vi "Teleop.vi"(10 "Match Info":T1={"Autonomous Elapsed Seconds"=0.0, "TeleOp Elapsed Seconds"=0.0, "Disabled Elapsed Seconds"=0.0, "Visited Autonomous"=FALSE, "Visited TeleOp"=FALSE, "Visited Disabled"=FALSE, "Autonomous Settings"={"Autonomous Style"=enum."Independent", "VI Refnum"=refnum}}, 11 "Call Context":T2) -> ()   [LabVIEW 2018]
doc: "This VI is called for each enabled TeleOp packet received from the DS. It is typically used to read from joysticks and other inputs and update I/O or setpoints for timed control loops. It should complete and return within 20 milliseconds or risk missing DS packets."
uses:
  <vilib>/Rock Robotics/WPI/DriverStation/WPI_DriverStationDerivedRobotMode.ctl
  <vilib>/Rock Robotics/WPI/DriverStation/WPI_DriverStationMatch Info.ctl
  <vilib>/Rock Robotics/WPI/ThirdParty/Phoenix-LabVIEW/Motor Controller/Controls/CTRE_Phoenix_MotorControl_ControlMode.ctl
  <vilib>/Rock Robotics/WPI/Utilities/WPI_GetSetVariantRefNum.vi
  <vilib>/Rock Robotics/Network Tables/NT Write Boolean.vi
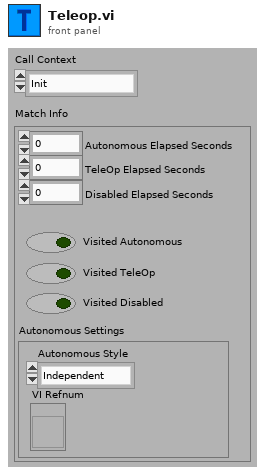
[diagram p1: front panel]
types:
  T1 = typedef "WPI_DriverStationMatch Info.ctl" = cluster{"Autonomous Elapsed Seconds":dbl, "TeleOp Elapsed Seconds":dbl, "Disabled Elapsed Seconds":dbl, "Visited Autonomous":bool, "Visited TeleOp":bool, "Visited Disabled":bool, "Autonomous Settings":cluster{"Autonomous Style":enum16{"Iterative", "Independent"}, "VI Refnum":refnum<vi>}}
  T2 = typedef "WPI_DriverStationDerivedRobotMode.ctl" = enum16{"Init", "Execute", "Stop"}
  T3 = enum16{"Low Ball", "Middle Ball", "High Ball", "High Hatch", "Middle Hatch", "Low Hatch", "Cargo Ball", "Ball Loading Station", "Ball Ground", "Reserve"}
  T4 = typedef "WPI_JoystickDevRef.ctl" = cluster{"Device":T5}
  T5 = typedef "WPI_JoystickDeviceEnum.ctl" = enum16{"USB 0", "USB 1", "USB 2", "USB 3", "USB 4", "USB 5"}
  T6 = cluster{"POVs[0]":i16, "POVs[1]":i16, "POVs[2]":i16, "POVs[3]":i16, "POVs[4]":i16, "POVs[5]":i16, "POVs[6]":i16, "POVs[7]":i16, "POVs[8]":i16}
  T7 = typedef "WPI_MotorControlDeviceRef.ctl" = cluster{"DeviceStatus":errorcluster, "Type":T8, "PWM":cluster{"PWM Channel":T9, "DeadBand":T10}, "CAN":cluster{"Device Number":u8, "SetOutput VI Ref":variant, "GetOutput VI Ref":variant, "Enable VI Ref":variant, "Disable VI Ref":variant, "Data":variant}, "Invert":bool, "DIO PWM":cluster{"PWM \"Enable\" Channel":T9, "DIOChannel":T11, "PWM Rate":dbl}}
  T8 = typedef "WPI_MotorControlType.ctl" = enum16{"PWM", "CAN", "DIO PWM"}
  T9 = typedef "FPGA_DIOPWMChannel.ctl" = enum8{"PWM 0", "PWM 1", "PWM 2", "PWM 3", "PWM 4", "PWM 5", "PWM 6", "PWM 7", "PWM 8", "PWM 9", "PWM MXP 0", "PWM MXP 1", "PWM MXP 2", "PWM MXP 3", "PWM MXP 4", "PWM MXP 5", "PWM MXP 6", "PWM MXP 7", "PWM MXP 8", "PWM MXP 9", "Invalid"}
  T10 = typedef "WPI_PWMDeadband.ctl" = cluster{"Name":string, "maxPositivePwm":i32, "minPositivePwm":i32, "centerPwm":i32, "maxNegativePwm":i32, "minNegativePwm":i32, "angularRange":u16}
  T11 = typedef "FPGA_DIOChannel.ctl" = enum8{"DIO 0", "DIO 1", "DIO 2", "DIO 3", "DIO 4", "DIO 5", "DIO 6", "DIO 7", "DIO 8", "DIO 9", "DIO MXP 0", "DIO MXP 1", "DIO MXP 2", "DIO MXP 3", "DIO MXP 4", "DIO MXP 5", "DIO MXP 6", "DIO MXP 7", "DIO MXP 8", "DIO MXP 9", "DIO MXP 10", "DIO MXP 11", "DIO MXP 12", "DIO MXP 13", "DIO MXP 14", "DIO MXP 15", "SPI Port CS1", "SPI Port CS2", "SPI Port CS3", "SPI Port MISO", "SPI Port MOSI", "Invalid"}
  T12 = typedef "CTRE_Phoenix_MotorControl_ControlMode.ctl" = u16
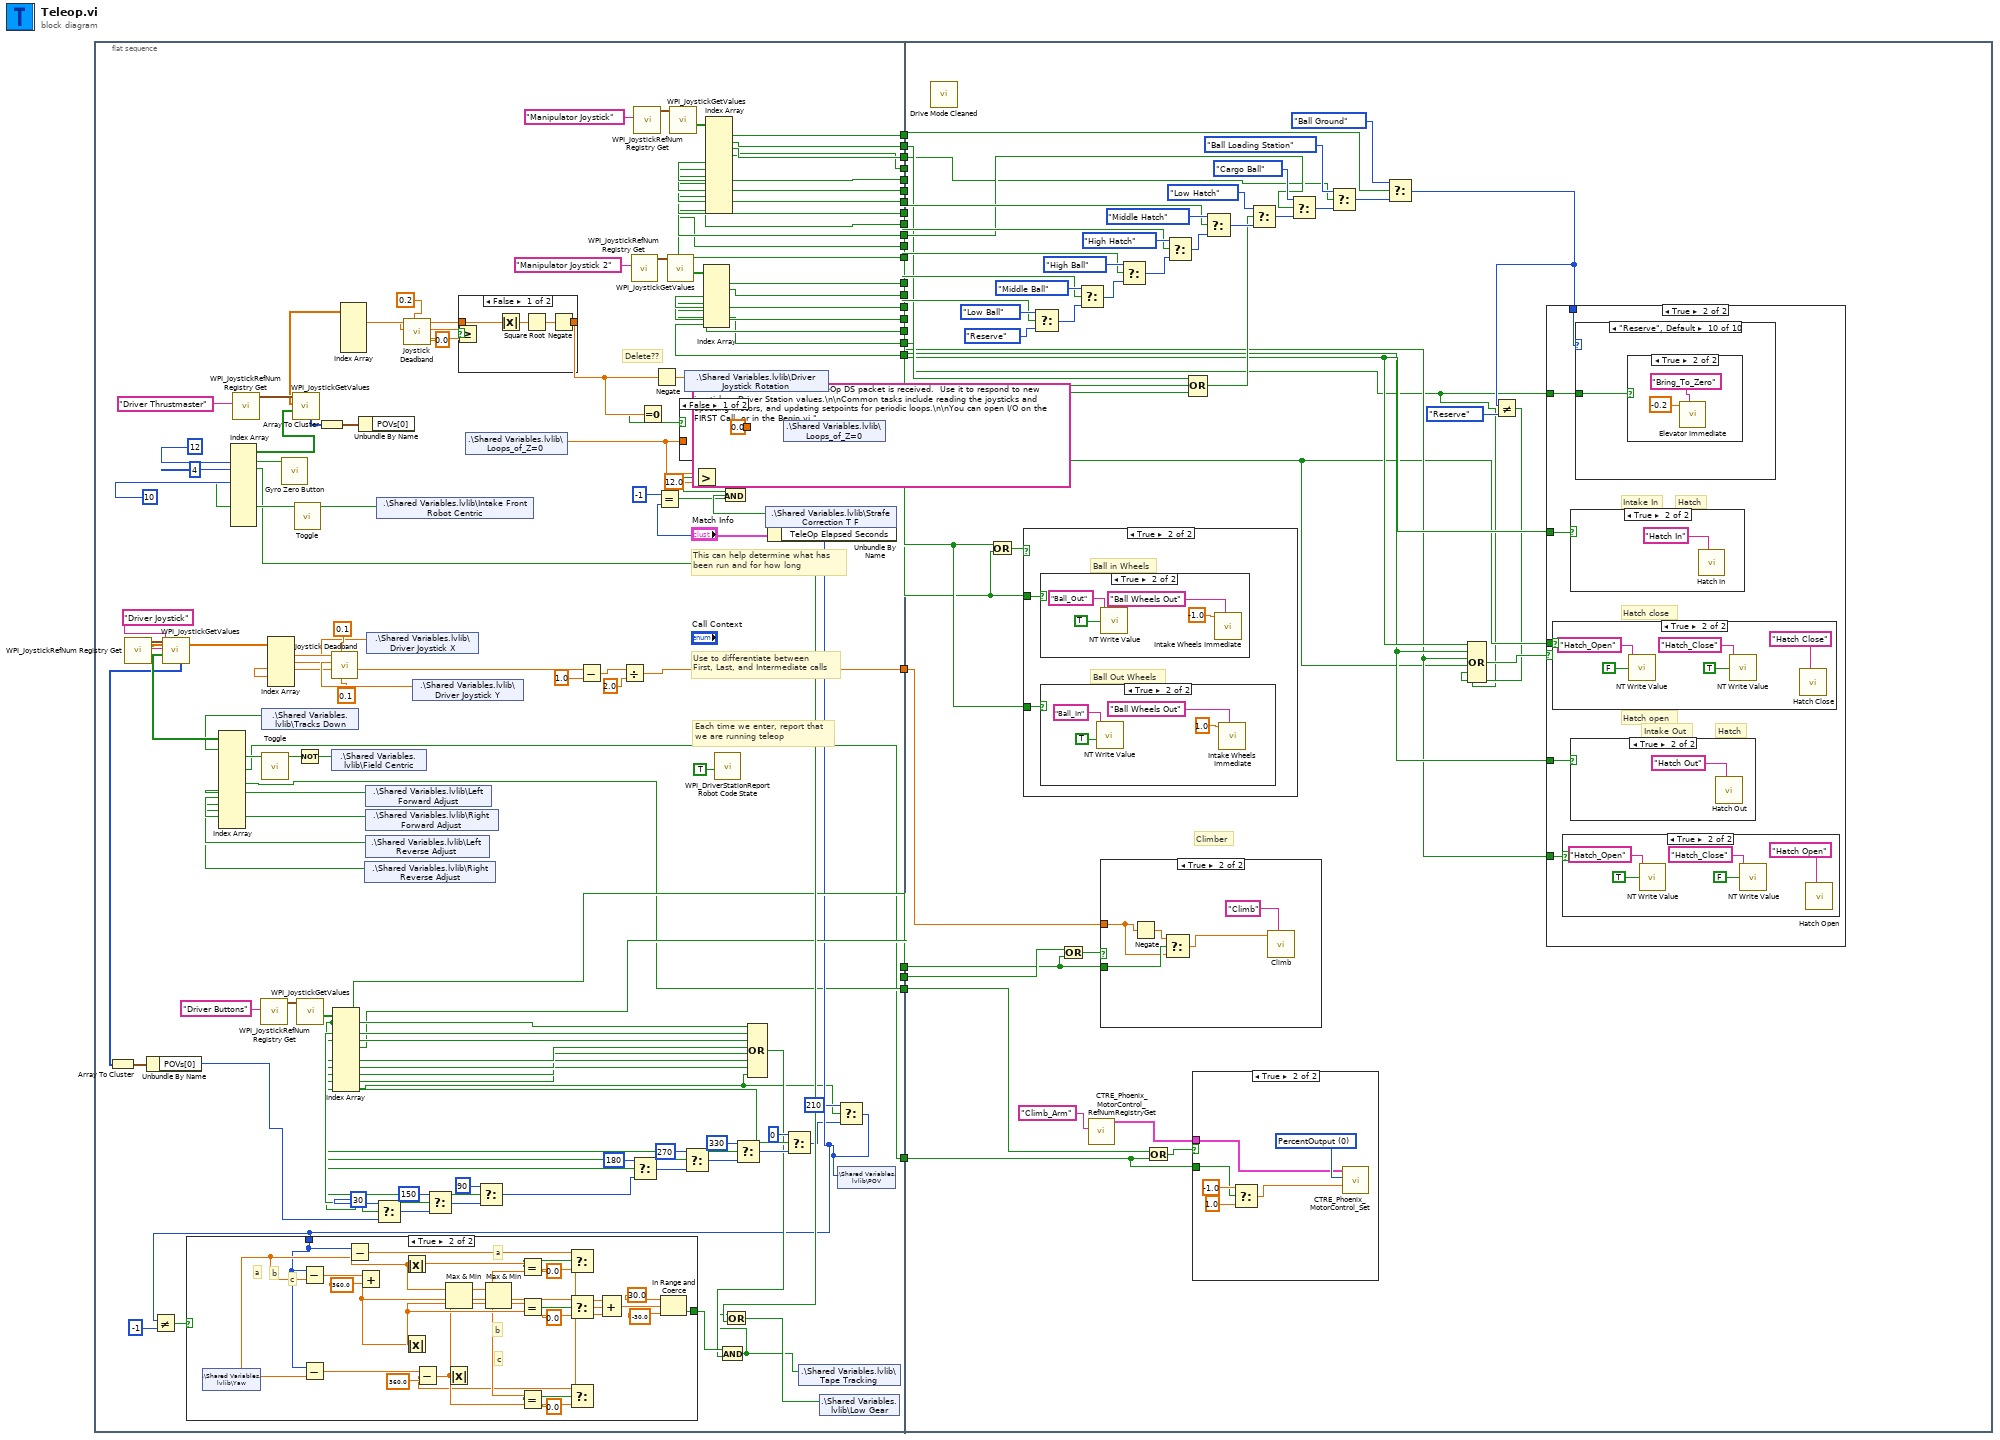
[diagram p0: block diagram]
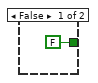
[diagram p2: hidden frame]
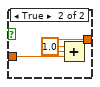
[diagram p3: hidden frame]
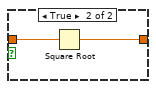
[diagram p4: hidden frame]
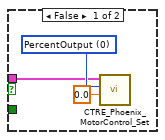
[diagram p5: hidden frame]
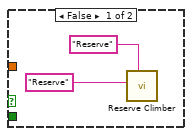
[diagram p6: hidden frame]
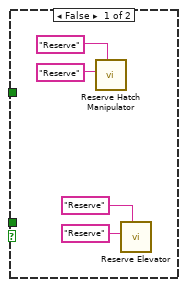
[diagram p7: hidden frame]
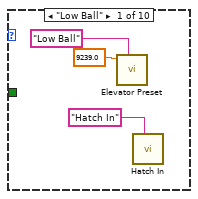
[diagram p8: hidden frame]
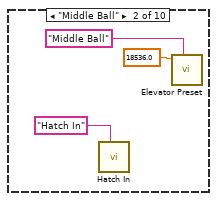
[diagram p9: hidden frame]
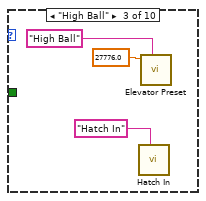
[diagram p10: hidden frame]
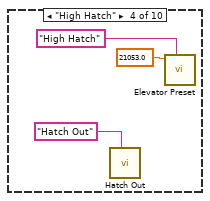
[diagram p11: hidden frame]
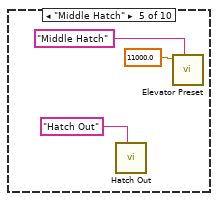
[diagram p12: hidden frame]
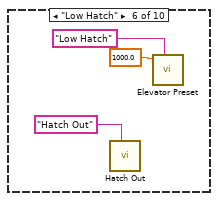
[diagram p13: hidden frame]
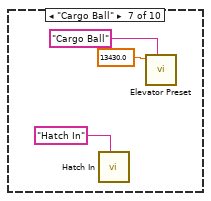
[diagram p14: hidden frame]
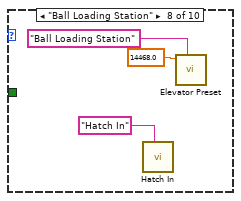
[diagram p15: hidden frame]
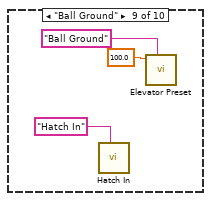
[diagram p16: hidden frame]
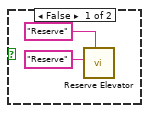
[diagram p17: hidden frame]
diagram:
  (unwired) "This VI is called each time a TeleOp DS packet is received.  Use it to respond to new joystick or Driver Station values.\n\nCommon tasks include reading the joysticks and updating motors, and updating setpoints for periodic loops.\n\nYou can open I/O on the FIRST Call, or in the Begin.vi."
  # "Each time we enter, report that\nwe are running teleop"
  # "Use to differentiate between\nFirst, Last, and Intermediate calls"
  # "This can help determine what has\nbeen run and for how long"
  n1 = flat-sequence {
    tunnel: [w43] -> w24
    tunnel: [w101] -> w23
    tunnel: [w100] -> w22
    tunnel: [w99] -> w21
    tunnel: [w98] -> w20
    tunnel: [w97] -> w19
    tunnel: [w96] -> w18
    tunnel: [w95] -> w17
    tunnel: [w94] -> w16
    tunnel: [w93] -> w15
    tunnel: [w92] -> w14
    tunnel: [w91] -> w13
    tunnel: [w90] -> w12
    tunnel: [w89] -> w11
    tunnel: [w88] -> w10
    tunnel: [w87] -> w9
    tunnel: [w86] -> w8
    tunnel: [w85] -> w7
    tunnel: [w84] -> w6
    tunnel: [w83] -> w5
    tunnel: [w46] -> w4
    tunnel: [w45] -> w3
    tunnel: [w29] -> w2
    tunnel: [w28] -> w1
    tunnel: w24 -> [w189]
    tunnel: w23 -> [w205]
    tunnel: w22 -> [w208]
    tunnel: w21 -> [w204]
    tunnel: w20 -> [w210]
    tunnel: w19 -> [w207]
    tunnel: w18 -> [w213]
    tunnel: w17 -> [w211]
    tunnel: w16 -> [w200]
    tunnel: w15 -> [w214]
    tunnel: w14 -> [w209]
    tunnel: w13 -> [w212]
    tunnel: w12 -> [w201]
    tunnel: w11 -> [w196]
    tunnel: w10 -> [_]
    tunnel: w9 -> [w199]
    tunnel: w8 -> [w197]
    tunnel: w7 -> [w198]
    tunnel: w6 -> [w187]
    tunnel: w5 -> [w203]
    tunnel: w4 -> [w191]
    tunnel: w3 -> [w190]
    tunnel: w2 -> [w183]
    tunnel: w1 -> [w182]
    frame #0 {
      # "Delete??"
      n2 = call <vilib>:"WPI_JoystickRefNum Registry Get.vi"("refnum name"="Driver Joystick") -> ("JoystickDevRef"=w143:T4)  [unwired: 1 in, 9 out]
      n3 = call <vilib>:"WPI_JoystickGetValues.vi"("JoystickDevRef"=w143) -> ("Buttons"=w129:bool[], "Axes"=w141:dbl[], "POVs"=w116:i16[])  [unwired: 6 in, 2 out]
      n4 = Array To Cluster(array=w116) -> (cluster=w117:T6)
      n5 = Unbundle By Name(w117) -> ("POVs[0]"=w27:i16)
      n6 = Index Array(array=w129) -> (element #1=w104:bool, element #2=w103:bool, element #4=w28:bool, element #6=w29:bool, element #7=w114:bool, element #8=w113:bool, element #9=w112:bool, element #10=w111:bool)  [unwired: 12 in, 4 out]
      n7 = call <vilib>:"WPI_JoystickRefNum Registry Get.vi"("refnum name"="Driver Thrustmaster") -> ("JoystickDevRef"=w131:T4)  [unwired: 9 in, 1 out]
      n8 = call <vilib>:"WPI_JoystickRefNum Registry Get.vi"("refnum name"="Driver Buttons") -> ("JoystickDevRef"=w81:T4)  [unwired: 1 in, 9 out]
      n9 = shared-variable ".\\Shared Variables.lvlib\\Tracks Down"(w104) -> ()  [unwired: 1 in, 1 out]
      n10 = call "Toggle.vi"("Input"=w103) -> ("Output"=w136:bool)  [unwired: 9 in, 1 out]
      n11 = Index Array(array=w141) -> (element #1=w135:dbl, element #2=w134:dbl, element #4=w105:dbl)  [unwired: 5 in, 2 out]
      n12 = call <vilib>:"WPI_JoystickGetValues.vi"("JoystickDevRef"=w131) -> ("Buttons"=w126:bool[], "Axes"=w130:dbl[], "POVs"=w118:i16[])  [unwired: 6 in, 2 out]
      n13 = Index Array(array=w126, index #1=12 ("index"), index #2=4 ("index"), index #4=10 ("index")) -> (element #1=w124:bool, element #2=w49:bool, element #4=w119:bool)  [unwired: 7 in, 7 out]
      n14 = call "Gyro Zero Button.vi"("Boolean"=w124) -> ()  [unwired: 11 in]
      n15 = call "Toggle.vi"("Input"=w119) -> ("Output"=w120:bool)  [unwired: 9 in, 1 out]
      n16 = Not(x=w136) -> (.not. x?=w133:bool)
      n17 = call <vilib>:"WPI_JoystickGetValues.vi"("JoystickDevRef"=w81) -> ("Buttons"=w41:bool[])  [unwired: 6 in, 4 out]
      n18 = Array To Cluster(array=w118) -> (cluster=w122:T6)
      n19 = call "Joystick Deadband.vi"("Z Deadband"=0.1, "X Y Deadband"=0.1, "Z"=w105, "Y"=w134, "X"=w135) -> ("Z Out"=w32:dbl, "Y Out"=w137:dbl, "X Out"=w109:dbl)  [unwired: 4 in]
      n20 = shared-variable ".\\Shared Variables.lvlib\\Field Centric"(w133) -> ()  [unwired: 1 in, 1 out]
      n21 = Index Array(array=w41) -> (element #1=w61:bool, element #2=w67:bool, element #3=w66:bool, element #4=w46:bool, element #5=w45:bool, element #6=w65:bool, element #7=w64:bool, element #8=w63:bool, element #9=w62:bool, element #10=w33:bool)  [unwired: 10 in]
      n22 = Index Array(array=w130) -> (element #1=w108:dbl)  [unwired: 5 in, 4 out]
      n23 = Unbundle By Name(w122) -> ()  [unwired: 1 out]
      n24 = shared-variable ".\\Shared Variables.lvlib\\Right Reverse Adjust"(w111) -> ()  [unwired: 1 in, 1 out]
      n25 = shared-variable ".\\Shared Variables.lvlib\\Left Forward Adjust"(w114) -> ()  [unwired: 1 in, 1 out]
      n26 = shared-variable ".\\Shared Variables.lvlib\\Right Forward Adjust"(w113) -> ()  [unwired: 1 in, 1 out]
      n27 = shared-variable ".\\Shared Variables.lvlib\\Left Reverse Adjust"(w112) -> ()  [unwired: 1 in, 1 out]
      n28 = shared-variable ".\\Shared Variables.lvlib\\Driver Joystick X"(w109) -> ()  [unwired: 1 in, 1 out]
      n29 = Select(t=i16 30, s=w61, f=w27) -> (s? t:f=w75:i16)
      n30 = shared-variable ".\\Shared Variables.lvlib\\Intake Front Robot Centric"(w120) -> ()  [unwired: 1 in, 1 out]
      n31 = call "Joystick Deadband.vi"("X Y Deadband"=0.2, "X"=w108) -> ("X Out"=w106:dbl)  [unwired: 7 in, 2 out]
      n32 = shared-variable ".\\Shared Variables.lvlib\\Driver Joystick Y"(w137) -> ()  [unwired: 1 in, 1 out]
      n33 = Select(t=i16 150, s=w67, f=w75) -> (s? t:f=w74:i16)
      n34 = Greater Or Equal?(x=w106, y=0.0) -> (x >= y?=w128:bool)
      n35 = case shown="False" w128 {
        tunnel: [w177 w181] -> w57
        tunnel: w106 -> [w176 w180]
        frame False {
          n36 = Absolute Value(x=w176) -> (abs(x)=w179:dbl)
          n37 = Square Root(x=w179) -> (sqrt(x)=w178:dbl)
          n38 = Negate(x=w178) -> (-x=w177:dbl)
        }
        frame True {
          n39 = Square Root(x=w180) -> (sqrt(x)=w181:dbl)
        }
      }
      n40 = shared-variable ".\\Shared Variables.lvlib\\Loops_of_Z=0"() -> (w53:dbl)  [unwired: 1 in, 1 out]
      n41 = Select(t=i16 90, s=w66, f=w74) -> (s? t:f=w42:i16)
      n42 = Subtract(x=w32, y=1.0) -> (x-y=w31:dbl)
      n43 = Divide(x=w31, y=2.0) -> (x/y=w43:dbl)
      n44 = call <vilib>:"WPI_JoystickRefNum Registry Get.vi"("refnum name"="Manipulator Joystick 2") -> ("JoystickDevRef"=w82:T4)  [unwired: 1 in, 9 out]
      n45 = Select(t=i16 180, s=w65, f=w42) -> (s? t:f=w72:i16)
      n46 = call <vilib>:"WPI_JoystickRefNum Registry Get.vi"("refnum name"="Manipulator Joystick") -> ("JoystickDevRef"=w139:T4)  [unwired: 1 in, 9 out]
      n47 = Equal To 0?(x=w57) -> (x = 0?=w56:bool)
      n48 = Negate(x=w57) -> (-x=w110:dbl)
      n49 = call <vilib>:"WPI_JoystickGetValues.vi"("JoystickDevRef"=w82) -> ("Buttons"=w39:bool[])  [unwired: 6 in, 4 out]
      n50 = call <vilib>:"WPI_JoystickGetValues.vi"("JoystickDevRef"=w139) -> ("Buttons"=w40:bool[])  [unwired: 6 in, 4 out]
      n51 = case shown="False" w56 {
        tunnel: w53 -> [_ w175]
        tunnel: [0.0 w173] -> w55
        frame False {
        }
        frame True {
          n52 = Add(x=1.0, y=w175) -> (x+y=w173:dbl)
        }
      }
      n53 = Select(t=i16 270, s=w64, f=w72) -> (s? t:f=w70:i16)
      n54 = shared-variable ".\\Shared Variables.lvlib\\Driver Joystick Rotation"(w110) -> ()  [unwired: 1 in, 1 out]
      n55 = Greater?(x=w53, y=12.0) -> (0:w54:bool)
      n56 = Index Array(array=w39) -> (element #1=w89:bool, element #2=w88:bool, element #3=w87:bool, element #4=w86:bool, element #5=w85:bool, element #6=w84:bool, element #7=w83:bool)  [unwired: 7 in]
      n57 = Index Array(array=w40) -> (element #1=w101:bool, element #2=w100:bool, element #3=w99:bool, element #4=w98:bool, element #5=w97:bool, element #6=w96:bool, element #7=w95:bool, element #8=w94:bool, element #9=w93:bool, element #10=w92:bool, element #11=w91:bool, element #12=w90:bool)  [unwired: 12 in]
      n58 = Select(t=i16 330, s=w63, f=w70) -> (s? t:f=w68:i16)
      n59 = Compound Arithmetic op=OR(w61, w67, w66, w65, w64, w63, w62, w33) -> (w50:bool)
      n60 = shared-variable ".\\Shared Variables.lvlib\\Loops_of_Z=0"(w55) -> ()  [unwired: 1 in, 1 out]
      n61 = Select(t=i16 0, s=w62, f=w68) -> (s? t:f=w35:i16)
      n62 = Select(t=i16 210, s=w33, f=w35) -> (s? t:f=w36:i16)
      n63 = Not Equal?(x=w36, y=i16 -1) -> (x != y?=w38:bool)
      n64 = case shown="True" w38 {
        tunnel: [FALSE w169] -> w51
        tunnel: w36 -> [_ w146]
        frame False {
        }
        frame True {
          # "c"
          # "b"
          # "a"
          # "c"
          # "b"
          # "a"
          n65 = shared-variable ".\\Shared Variables.lvlib\\Yaw"() -> (w147:dbl)  [unwired: 1 in, 1 out]
          n66 = Subtract(x=w146, y=w147) -> (x-y=w168:dbl)
          n67 = Subtract(x=w146, y=w147) -> (x-y=w166:dbl)
          n68 = Subtract(x=w146, y=w147) -> (x-y=w157:dbl)
          n69 = Add(x=w168, y=360.0) -> (x+y=w158:dbl)
          n70 = Absolute Value(x=w157) -> (abs(x)=w163:dbl)
          n71 = Absolute Value(x=w158) -> (abs(x)=w162:dbl)
          n72 = Subtract(x=w166, y=360.0) -> (x-y=w156:dbl)
          n73 = Max & Min(x=w163, y=w162) -> (min(x,y)=w164:dbl)  [unwired: 1 out]
          n74 = Absolute Value(x=w156) -> (abs(x)=w160:dbl)
          n75 = Max & Min(x=w164, y=w160) -> (min(x,y)=w161:dbl)  [unwired: 1 out]
          n76 = Equal?(x=w163, y=w161) -> (x = y?=w155:bool)
          n77 = Equal?(x=w161, y=w162) -> (x = y?=w159:bool)
          n78 = Equal?(x=w161, y=w160) -> (x = y?=w154:bool)
          n79 = Select(t=w157, s=w155, f=0.0) -> (s? t:f=w150:dbl)
          n80 = Select(t=w158, s=w159, f=0.0) -> (s? t:f=w149:dbl)
          n81 = Select(t=w156, s=w154, f=0.0) -> (s? t:f=w148:dbl)
          n82 = Compound Arithmetic op=ADD(w150, w149, w148) -> (w145:dbl)
          n83 = In Range and Coerce(upper limit=30.0, x=w145, lower limit=-30.0) -> (In Range?=w169:bool)  [unwired: 1 out]
        }
      }
      n84 = Equal?(x=i16 -1, y=w36) -> (x = y?=w58:bool)
      n85 = And(x=w54, y=w58) -> (x .and. y?=w59:bool)
      n86 = Compound Arithmetic op=AND(w51, w50) -> (w47:bool)
      n87 = Or(x=w47, y=w49) -> (x .or. y?=w48:bool)
      n88 = shared-variable ".\\Shared Variables.lvlib\\Strafe Correction T F"(w59) -> ()  [unwired: 1 in, 1 out]
      n89 = shared-variable ".\\Shared Variables.lvlib\\Tape Tracking"(w47) -> ()  [unwired: 1 in, 1 out]
      n90 = shared-variable ".\\Shared Variables.lvlib\\Low Gear"(w48) -> ()  [unwired: 1 in, 1 out]
      n91 = shared-variable ".\\Shared Variables.lvlib\\POV"(w36) -> ()  [unwired: 1 in, 1 out]
    }
    frame #1 {
      # "Climber"
      n92 = call "Drive Mode Cleaned.vi"() -> ()  [unwired: 12 in]
      n93 = Or(x=w201, y=w200) -> (x .or. y?=w202:bool)
      n94 = case shown="True" w202 {
        tunnel: w201 -> [_ w310]
        tunnel: w200 -> [_ w309]
        frame False {
          n95 = call-poly <vilib>:"NT Write Value.vi"("Boolean"=FALSE, "Name"="Ball_Out") -> ()  [unwired: 9 in, 1 out]
          n96 = call "Reserve Intake.vi"("Description"="Reserve", "Command Name"="Reserve") -> ()  [unwired: 9 in, 1 out]
          n97 = call-poly <vilib>:"NT Write Value.vi"("Boolean"=FALSE, "Name"="Ball_In") -> ()  [unwired: 9 in, 1 out]
        }
        frame True {
          # "Ball in Wheels"
          # "Ball Out Wheels"
          n98 = case shown="True" w309 {
            frame False {
            }
            frame True {
              n99 = call-poly <vilib>:"NT Write Value.vi"("Boolean"=TRUE, "Name"="Ball_Out") -> ()  [unwired: 9 in, 1 out]
              n100 = call "Intake Wheels Immediate.vi"("Description"="Ball Wheels Out", "Setpoint"=-1.0) -> ()  [unwired: 9 in, 1 out]
            }
          }
          n101 = case shown="True" w310 {
            frame False {
            }
            frame True {
              n102 = call-poly <vilib>:"NT Write Value.vi"("Boolean"=TRUE, "Name"="Ball_In") -> ()  [unwired: 9 in, 1 out]
              n103 = call "Intake Wheels Immediate.vi"("Description"="Ball Wheels Out", "Setpoint"=1.0) -> ()  [unwired: 9 in, 1 out]
            }
          }
        }
      }
      n104 = Select(t=T3."Low Ball" ("Enum"), s=w210, f=T3."Reserve" ("Enum")) -> (s? t:f=w232:T3)
      n105 = Or(x=w191, y=w190) -> (x .or. y?=w192:bool)
      n106 = Select(t=T3."Middle Ball" ("Enum"), s=w211, f=w232) -> (s? t:f=w231:T3)
      n107 = call <vilib>:"CTRE_Phoenix_MotorControl_RefNumRegistryGet.vi"("refnum name"="Climb_Arm") -> ("PhoenixMotorControlDevRef"=w185:T7)  [unwired: 9 in, 1 out]
      n108 = case shown="True" w192 {
        tunnel: w190 -> [_ w247]
        tunnel: w189 -> [_ w245]
        frame False {
          n109 = call "Reserve Climber.vi"("Description"="Reserve", "Command Name"="Reserve" ("Description")) -> ()  [unwired: 9 in, 1 out]
        }
        frame True {
          n110 = Negate(x=w245) -> (-x=w246:dbl)
          n111 = Select(t=w246, s=w247, f=w245) -> (s? t:f=w244:dbl)
          n112 = call "Climb.vi"("Description"="Climb", "Setpoint"=w244) -> ()  [unwired: 9 in, 1 out]
        }
      }
      n113 = Select(t=T3."High Ball" ("Enum"), s=w212, f=w231) -> (s? t:f=w230:T3)
      n114 = Or(x=w183, y=w182) -> (x .or. y?=w184:bool)
      n115 = Select(t=T3."High Hatch" ("Enum"), s=w214, f=w230) -> (s? t:f=w229:T3)
      n116 = Compound Arithmetic op=OR(w208, w207, w203) -> (w206:bool)
      n117 = case shown="True" w184 {
        tunnel: w185 -> [w233 w236]
        tunnel: w182 -> [_ w238]
        frame False {
          w235 = T12 0 items=["PercentOutput"=0, "Position"=1, "Velocity"=2, "Current"=3, "Follower"=5, "MotionProfile"=6, "MotionMagic"=7, "MotionProfileArc"=10, "Disabled"=15] ("Control Mode")
          n118 = call <vilib>:"CTRE_Phoenix_MotorControl_Set.vi"("Output"=0.0, "Control Mode"=w235, "PhoenixMotorControlDevRef"=w233) -> ()  [unwired: 7 in, 2 out]
        }
        frame True {
          w241 = T12 0 items=["PercentOutput"=0, "Position"=1, "Velocity"=2, "Current"=3, "Follower"=5, "MotionProfile"=6, "MotionMagic"=7, "MotionProfileArc"=10, "Disabled"=15] ("Control Mode")
          n119 = Select(t=-1.0, s=w238, f=1.0) -> (s? t:f=w237:dbl)
          n120 = call <vilib>:"CTRE_Phoenix_MotorControl_Set.vi"("Output"=w237, "Control Mode"=w241, "PhoenixMotorControlDevRef"=w236) -> ()  [unwired: 7 in, 2 out]
        }
      }
      n121 = Select(t=T3."Middle Hatch" ("Enum"), s=w213, f=w229) -> (s? t:f=w228:T3)
      n122 = Select(t=T3."Low Hatch" ("Enum"), s=w206, f=w228) -> (s? t:f=w227:T3)
      n123 = Select(t=T3."Cargo Ball" ("Enum"), s=w209, f=w227) -> (s? t:f=w226:T3)
      n124 = Select(t=T3."Ball Loading Station" ("Enum"), s=w204, f=w226) -> (s? t:f=w216:T3)
      n125 = Select(t=T3."Ball Ground" ("Enum"), s=w205, f=w216) -> (s? t:f=w194:T3)
      n126 = Not Equal?(x=w194, y=T3."Reserve" ("Enum")) -> (x != y?=w188:bool)
      n127 = Compound Arithmetic op=OR(w199, w198, w197, w196, w188, w187) -> (w195:bool)
      n128 = case shown="True" w195 {
        tunnel: w199 -> [_ w258]
        tunnel: w197 -> [_ w257]
        tunnel: w198 -> [_ w256]
        tunnel: w196 -> [_ w255]
        tunnel: w194 -> [_ w254]
        tunnel: w187 -> [_ w253]
        frame False {
          n129 = call "Reserve Hatch Manipulator.vi"("Description"="Reserve", "Command Name"="Reserve") -> ()  [unwired: 9 in, 1 out]
          n130 = call "Reserve Elevator.vi"("Description"="Reserve", "Command Name"="Reserve") -> ()  [unwired: 9 in, 1 out]
        }
        frame True {
          # "Hatch"
          # "Hatch"
          # "Hatch open"
          # "Hatch close"
          # "Intake In"
          # "Intake Out"
          n131 = case shown="True" w255 {
            frame False {
            }
            frame True {
              n132 = call-poly <vilib>:"NT Write Value.vi"("Boolean"=FALSE, "Name"="Hatch_Open") -> ()  [unwired: 9 in, 1 out]
              n133 = call-poly <vilib>:"NT Write Value.vi"("Boolean"=TRUE, "Name"="Hatch_Close") -> ()  [unwired: 9 in, 1 out]
              n134 = call "Hatch Close.vi"("Description"="Hatch Close") -> ()  [unwired: 10 in, 1 out]
            }
          }
          n135 = case shown="True" w257 {
            frame False {
            }
            frame True {
              n136 = call-poly <vilib>:"NT Write Value.vi"("Boolean"=TRUE, "Name"="Hatch_Open") -> ()  [unwired: 9 in, 1 out]
              n137 = call-poly <vilib>:"NT Write Value.vi"("Boolean"=FALSE, "Name"="Hatch_Close") -> ()  [unwired: 9 in, 1 out]
              n138 = call "Hatch Open.vi"("Description"="Hatch Open") -> ()  [unwired: 10 in, 1 out]
            }
          }
          n139 = case shown="True" w258 {
            frame False {
            }
            frame True {
              n140 = call "Hatch In.vi"("Description"="Hatch In") -> ()  [unwired: 10 in, 1 out]
            }
          }
          n141 = case shown="True" w256 {
            frame False {
            }
            frame True {
              n142 = call "Hatch Out.vi"("Description"="Hatch Out") -> ()  [unwired: 10 in, 1 out]
            }
          }
          n143 = case shown="\"Reserve\", Default" w254 {
            tunnel: w253 -> [_ _ _ _ _ _ _ _ _ w286]
            frame "Low Ball" {
              n144 = call "Elevator Preset.vi"("Description"="Low Ball", "Position"=9239.0) -> ()  [unwired: 9 in, 1 out]
              n145 = call "Hatch In.vi"("Description"="Hatch In") -> ()  [unwired: 10 in, 1 out]
            }
            frame "Middle Ball" {
              n146 = call "Hatch In.vi"("Description"="Hatch In") -> ()  [unwired: 10 in, 1 out]
              n147 = call "Elevator Preset.vi"("Description"="Middle Ball", "Position"=18536.0) -> ()  [unwired: 9 in, 1 out]
            }
            frame "High Ball" {
              n148 = call "Hatch In.vi"("Description"="Hatch In") -> ()  [unwired: 10 in, 1 out]
              n149 = call "Elevator Preset.vi"("Description"="High Ball", "Position"=27776.0) -> ()  [unwired: 9 in, 1 out]
            }
            frame "High Hatch" {
              n150 = call "Hatch Out.vi"("Description"="Hatch Out") -> ()  [unwired: 10 in, 1 out]
              n151 = call "Elevator Preset.vi"("Description"="High Hatch", "Position"=21053.0) -> ()  [unwired: 9 in, 1 out]
            }
            frame "Middle Hatch" {
              n152 = call "Hatch Out.vi"("Description"="Hatch Out") -> ()  [unwired: 10 in, 1 out]
              n153 = call "Elevator Preset.vi"("Description"="Middle Hatch", "Position"=11000.0) -> ()  [unwired: 9 in, 1 out]
            }
            frame "Low Hatch" {
              n154 = call "Hatch Out.vi"("Description"="Hatch Out") -> ()  [unwired: 10 in, 1 out]
              n155 = call "Elevator Preset.vi"("Description"="Low Hatch", "Position"=1000.0) -> ()  [unwired: 9 in, 1 out]
            }
            frame "Cargo Ball" {
              n156 = call "Hatch In.vi"("Description"="Hatch In") -> ()  [unwired: 10 in, 1 out]
              n157 = call "Elevator Preset.vi"("Description"="Cargo Ball", "Position"=13430.0) -> ()  [unwired: 9 in, 1 out]
            }
            frame "Ball Loading Station" {
              n158 = call "Hatch In.vi"("Description"="Hatch In") -> ()  [unwired: 10 in, 1 out]
              n159 = call "Elevator Preset.vi"("Description"="Ball Loading Station", "Position"=14468.0) -> ()  [unwired: 9 in, 1 out]
            }
            frame "Ball Ground" {
              n160 = call "Hatch In.vi"("Description"="Hatch In") -> ()  [unwired: 10 in, 1 out]
              n161 = call "Elevator Preset.vi"("Description"="Ball Ground", "Position"=100.0) -> ()  [unwired: 9 in, 1 out]
            }
            frame "Reserve", Default {
              n162 = case shown="True" w286 {
                frame False {
                  n163 = call "Reserve Elevator.vi"("Description"="Reserve", "Command Name"="Reserve") -> ()  [unwired: 9 in, 1 out]
                }
                frame True {
                  n164 = call "Elevator Immediate.vi"("Description"="Bring_To_Zero", "Speed"=-0.2) -> ()  [unwired: 9 in, 1 out]
                }
              }
            }
          }
        }
      }
    }
  }
  n165 = call <vilib>:"WPI_DriverStationReport Robot Code State.vi"("TeleOp"=TRUE ("Autonomous")) -> ()  [unwired: 10 in, 1 out]
  n166 = Unbundle By Name("Match Info") -> ()  [unwired: 1 out]
